vi "niDTS WLAN INSTR RX Configure Basic.vi"(8 "error in (no error)":errorcluster, 11 "niDTS WLAN INSTR RX in":refnum<class "niDTS WLAN INSTR RX.lvclass">) -> (0 "error out":errorcluster, 3 "niDTS WLAN INSTR RX out":refnum<class "niDTS WLAN INSTR RX.lvclass">)   [LabVIEW 2015, in "niDTS WLAN.lvlib" / "niDTS WLAN INSTR RX.lvclass"]
doc: "Sets:\n\n* WlanStandard\n* ChannelBandwidth\n* PowerLevel\n* CarrierFrequency\n* IdleTime\n* NumberOfPackets"
uses:
  niDTS WLAN INSTR RX.lvclass
  niDTS WLAN INSTR RX.lvclass/niDTS WLAN INSTR RX.ctl
  RiviInstDriver/niRfsgWlan/Objects/niRfsgWlan.lvclass
  niDTS WLAN.lvlib
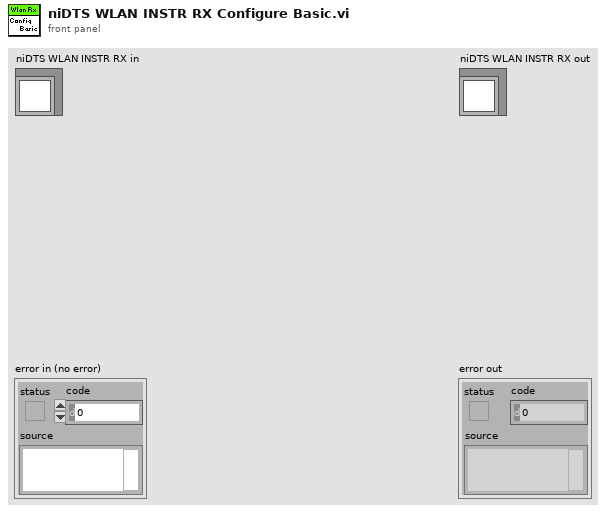
[diagram p1: front panel]
types:
  T1 = typedef "niRfsgWlan.lvclass/niRfsgWlan INC Handle.ctl" = refnum<data-value>
  T2 = typedef "niDTS WLAN.lvlib/niDTS WLAN INC Standard.ctl" = enum16{"802.11 b DSSS", "802.11 a/g OFDM", "802.11 n HT", "802.11 ac VHT"}
  T3 = typedef "niDTS WLAN.lvlib/niDTS WLAN INC CH BW.ctl" = enum16{"20 MHz", "40 MHz", "80 MHz", "160 MHz"}
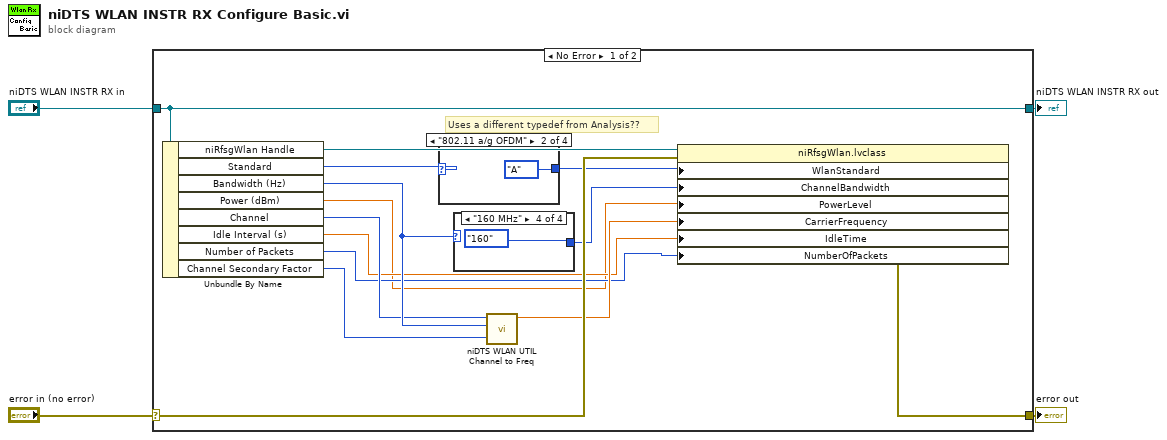
[diagram p0: block diagram]
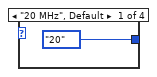
[diagram p2: hidden frame]
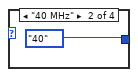
[diagram p3: hidden frame]
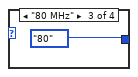
[diagram p4: hidden frame]
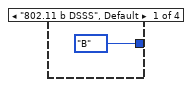
[diagram p5: hidden frame]
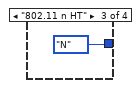
[diagram p6: hidden frame]
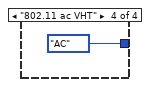
[diagram p7: hidden frame]
diagram:
  n1 = case shown="No Error" "error in (no error)" {
    selector: "error in (no error)" -> [w13 w28]
    tunnel: [w10 w28] -> w3
    tunnel: [w18 w27] -> w1
    tunnel: "niDTS WLAN INSTR RX in" -> [w18 w27]
    frame No Error {
      # "Uses a different typedef from Analysis??"
      n2 = Unbundle By Name(w18) -> ("niRfsgWlan Handle"=w14:T1, "Standard"=w17:T2, "Bandwidth (Hz)"=w16:T3, "Power (dBm)"=w6:dbl, "Channel"=w15:i32, "Idle Interval (s)"=w9:dbl, "Number of Packets"=w8:i32, "Channel Secondary Factor"=w7:enum16{"-1", "1", "0"})
      n3 = case shown="\"802.11 a/g OFDM\"" w17 {
        tunnel: [enum16{"A", "B", "G", "N", "AC"}."B" ("CONFigure:RFSG:WLAN:WlanStandard") enum16{"A", "B", "G", "N", "AC"}."A" ("CONFigure:RFSG:WLAN:WlanStandard") enum16{"A", "B", "G", "N", "AC"}."N" ("CONFigure:RFSG:WLAN:WlanStandard") enum16{"A", "B", "G", "N", "AC"}."AC" ("CONFigure:RFSG:WLAN:WlanStandard")] -> w12
        frame "802.11 b DSSS", Default {
        }
        frame "802.11 a/g OFDM" {
        }
        frame "802.11 n HT" {
        }
        frame "802.11 ac VHT" {
        }
      }
      n4 = case shown="\"160 MHz\"" w16 {
        tunnel: [enum16{"5", "10", "20", "40", "80", "160"}."20" ("SOURce:RFSG:WLAN:ChannelBandwidth") enum16{"5", "10", "20", "40", "80", "160"}."40" ("SOURce:RFSG:WLAN:ChannelBandwidth") enum16{"5", "10", "20", "40", "80", "160"}."80" ("SOURce:RFSG:WLAN:ChannelBandwidth") enum16{"5", "10", "20", "40", "80", "160"}."160" ("SOURce:RFSG:WLAN:ChannelBandwidth")] -> w5
        frame "20 MHz", Default {
        }
        frame "40 MHz" {
        }
        frame "80 MHz" {
        }
        frame "160 MHz" {
        }
      }
      n5 = call "niDTS WLAN UTIL Channel to Freq.vi"("secondary factor"=w7, "CH BW"=w16, "Channel"=w15) -> ("Center Frequency (Hz)"=w11:dbl)  [unwired: 6 in, 2 out]
      n6 = property class="niRfsgWlan.lvclass"(reference=w14, error in=w13, "WlanStandard"=w12, "ChannelBandwidth"=w5, "PowerLevel"=w6, "CarrierFrequency"=w11, "IdleTime"=w9, "NumberOfPackets"=w8) -> (error out=w10:errorcluster)  [unwired: 1 out]
    }
    frame Error {
    }
  }
  "error out" <- w3
  "niDTS WLAN INSTR RX out" <- w1
